vi "例程11-全局变量的使用2.vi"() -> ()   [LabVIEW 2016]
panel:
  out "数值":i32
  in  "总开关":bool
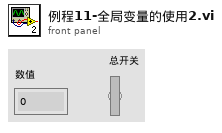
[diagram p1: front panel]
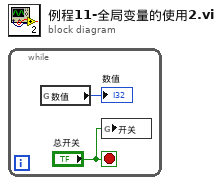
[diagram p0: block diagram]
diagram:
  n1 = while {
    stop <- "总开关" stop-if-true
    n2 = global read "例程11-全局.vi" "数值"() -> (→"数值":i32)
    n3 = global write "例程11-全局.vi" "开关"("总开关") -> ()
  }
